vi "CorectionCurve.vi"(9 "Data from power sumply":dbl[](array[numeric]), 10 "Data calibration multimeter":dbl[](array[numeric]), 11 "Data ethalon":dbl[](array[numeric])) -> (0 "XY Graph":cluster{"Data from power sumply ":dbl[], dbl[]}(graph), 1 "Relative fault":dbl[](array[numeric]), 2 "Absolute fault":dbl[](array[numeric]), 3 "Correction":dbl[](array[numeric]))   [LabVIEW 2022 SP3]
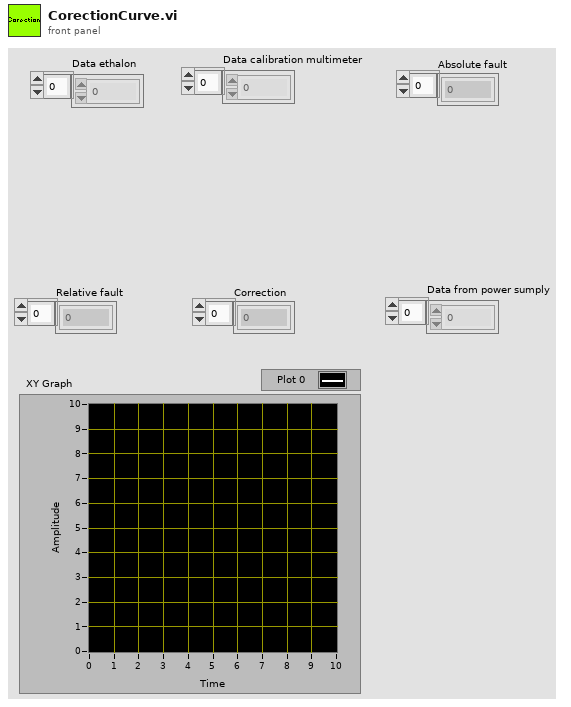
[diagram p1: front panel]
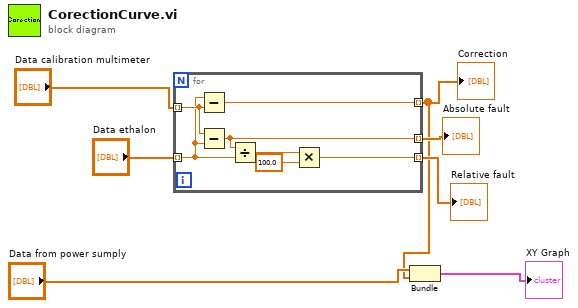
[diagram p0: block diagram]
diagram:
  n1 = for {
    tunnel: "Data calibration multimeter" -> [w14] mode=indexing
    tunnel: "Data ethalon" -> [w12] mode=indexing
    tunnel: [w13] -> w5 mode=indexing
    tunnel: [w9] -> w4 mode=indexing
    tunnel: [w8] -> w2 mode=indexing
    n2 = Subtract(x=w12, y=w14) -> (x-y=w8:dbl)
    n3 = Subtract(x=w14, y=w12) -> (x-y=w13:dbl)
    n4 = Divide(x=w13, y=w12) -> (x/y=w11:dbl)
    n5 = Multiply(x=w11, y=100.0) -> (x*y=w9:dbl)
  }
  "Absolute fault" <- w5
  "Relative fault" <- w4
  "Correction" <- w2
  n6 = Bundle("Data from power sumply"="Data from power sumply", w2) -> (→"XY Graph":cluster{"Data from power sumply ":dbl[], dbl[]})  [unwired: 1 in]
